vi "Binomial Noise.vi"(7 "initialize?":bool=TRUE, 8 "seed":i32=-1, 9 "trial probability":dbl=0.5 format="%.2f", 10 "trials":i32=1, 11 "samples":i32=128) -> (0 "error":i32, 3 "binomial noise":u32[](array[numeric]))   [LabVIEW 2020, in "NI_AALBase.lvlib"]
doc: "Generates a binomially-distributed, pseudorandom pattern whose values are the number of occurrences of an event, given the probability of that event occurring and the number of trials."
uses:
  NI_AALBase.lvlib
  <resource>/lvanlys.dll
panel:
  # "Binomial Noise"
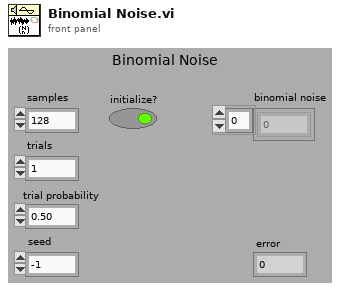
[diagram p1: front panel]
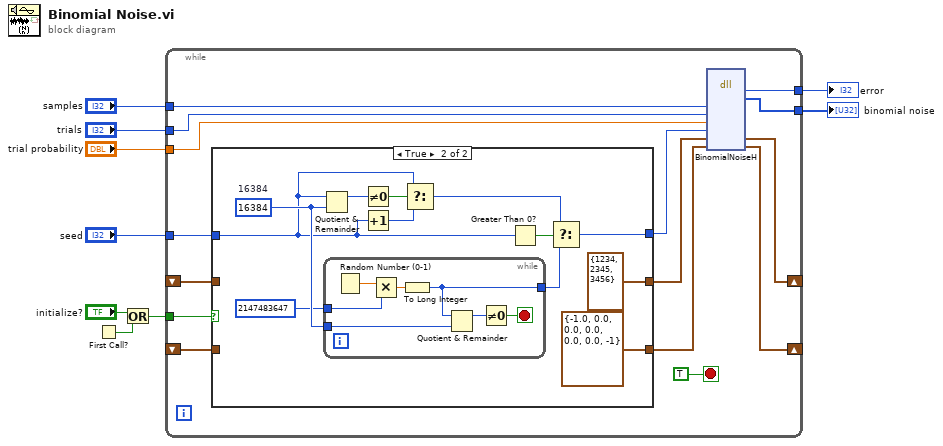
[diagram p0: block diagram]
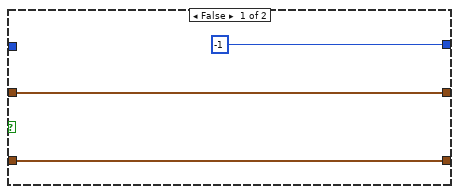
[diagram p2: hidden frame]
diagram:
  n1 = First Call?() -> (First Call?: T/F=w3:bool)
  n2 = Or(x="initialize?", y=w3) -> (x .or. y?=w2:bool)
  n3 = while {
    tunnel: [w21] -> w9
    tunnel: "seed" -> [w18]
    tunnel: "trials" -> [w24]
    tunnel: "samples" -> [w23]
    shift-right: [w10] -> _
    shift-left: _ -> [w19]
    shift-right: [w15] -> _
    shift-left: _ -> [w17]
    tunnel: w2 -> [w20]
    tunnel: "trial probability" -> [w12]
    tunnel: [w11] -> w1
    stop <- TRUE stop-if-true
    n4 = case shown="True" w20 {
      tunnel: w19 -> [w27 _]
      tunnel: [w27 cluster{"xSeed":i32, "ySeed":i32, "zSeed":i32} {"xSeed"=1234, "ySeed"=2345, "zSeed"=3456} ("RNGState")] -> w14
      tunnel: [-1 ("seed") w28] -> w13
      tunnel: w18 -> [_ w29]
      tunnel: [w26 cluster{dbl, dbl, dbl, dbl, dbl, dbl, i32} {-1.0, 0.0, 0.0, 0.0, 0.0, 0.0, -1}] -> w16
      tunnel: w17 -> [w26 _]
      frame False {
      }
      frame True {
        w31 = 16384  # 16384
        n5 = Quotient & Remainder(x=w29, y=w31) -> (x-y*floor(x/y)=w36:i32)  [unwired: 1 out]
        n6 = while {
          tunnel: [w44] -> w32
          tunnel: w31 -> [w43]
          tunnel: 2147483647 ("x") -> [w40]
          stop <- w41 stop-if-true
          n7 = Random Number (0-1)() -> (number: 0 to 1=w45:dbl)
          n8 = Multiply(x=w45, y=w40) -> (x*y=w46:dbl)
          n9 = To Long Integer(number=w46) -> (32bit integer=w44:i32)
          n10 = Quotient & Remainder(x=w44, y=w43) -> (x-y*floor(x/y)=w42:i32)  [unwired: 1 out]
          n11 = Not Equal To 0?(x=w42) -> (x != 0?=w41:bool)
        }
        n12 = Not Equal To 0?(x=w36) -> (x != 0?=w35:bool)
        n13 = Increment(x=w29) -> (x+1=w34:i32)
        n14 = Select(t=w29, s=w35, f=w34) -> (s? t:f=w33:i32)
        n15 = Greater Than 0?(x=w29) -> (x > 0?=w37:bool)
        n16 = Select(t=w33, s=w37, f=w32) -> (s? t:f=w28:i32)
      }
    }
    n17 = dll-call lib="C:/Program Files (x86)/National Instruments/LabVIEW 2020/resource/lvanlys.*" fn="BinomialNoiseH"("size"=w23, "numTrials"=w24, "trialProb"=w12, "theSeed"=w13, "rngState"=w14, "binomialState"=w16) -> ("return type"=w21:i32, "xH"=w11:u32[], "rngState"=w10:cluster{"xSeed":i32, "ySeed":i32, "zSeed":i32}, "binomialState"=w15:cluster{dbl, dbl, dbl, dbl, dbl, dbl, i32})  [unwired: 7 in, 3 out]
  }
  "error" <- w9
  "binomial noise" <- w1
